vi "Manage Waypoint Shape.vi"(4 "Valid Path?":bool=TRUE, 5 "Draw Arrow":bool, 6 "Coords":cluster{"x":dbl, "y":dbl}, 7 "Drawing Options":T1, 8 "Operation":enum16{"Draw", "Pt Test"}(ring), 9 "new picture in":picture, 10 "Waypoint Position (ft)":cluster{"x":dbl, "y":dbl, "th":dbl}, 11 "Pict Ref":refnum<vi>) -> (0 "Pt Test Results":enum16{"Miss", "Rect Hit", "Arrow Hit"}(ring), 1 "new picture out":picture)   [LabVIEW 2023]
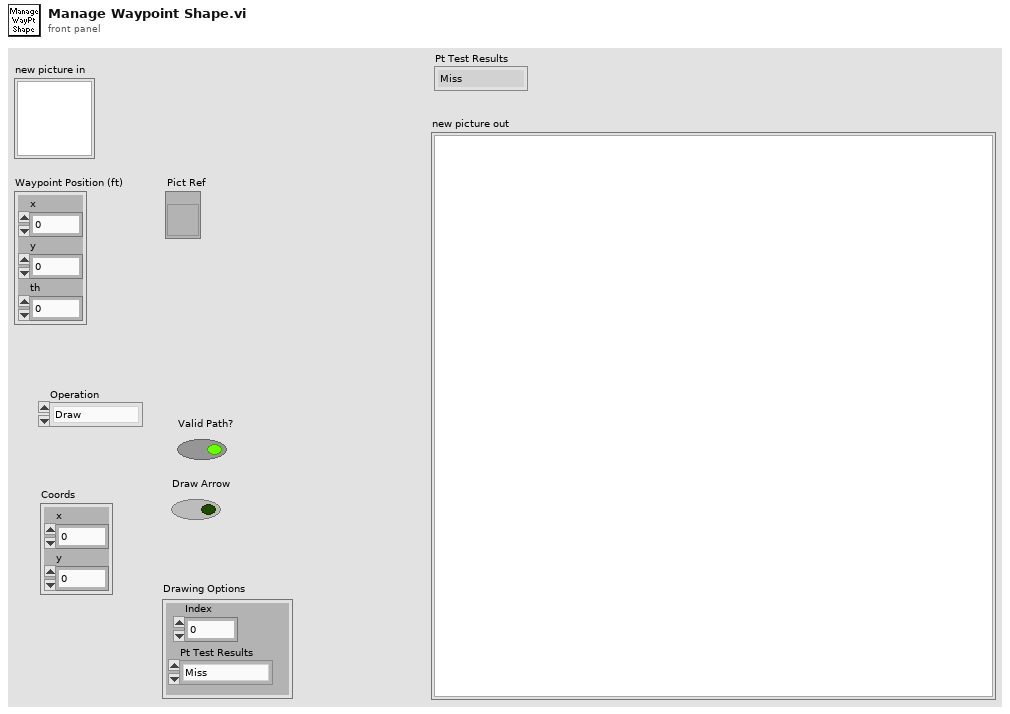
[diagram p1: front panel]
types:
  T1 = cluster{"Index":u32, "Pt Test Results":enum16{"Miss", "Rect Hit", "Arrow Hit"}}
  T2 = typedef "LVPositionTypeDef.ctl" = cluster{"Left":i32, "Top":i32}
  T3 = typedef "LVBoundsTypeDef.ctl" = cluster{"Width":u32, "Height":u32}
  T4 = cluster{"horizontal":enum16{"left", "center", "right"}, "vertical":enum16{"top", "center", "bottom"}}
  T5 = cluster{"Width":u16, "Style":enum32{"Solid", "Dash", "Dot", "DashDot", "DashDotDot"}}
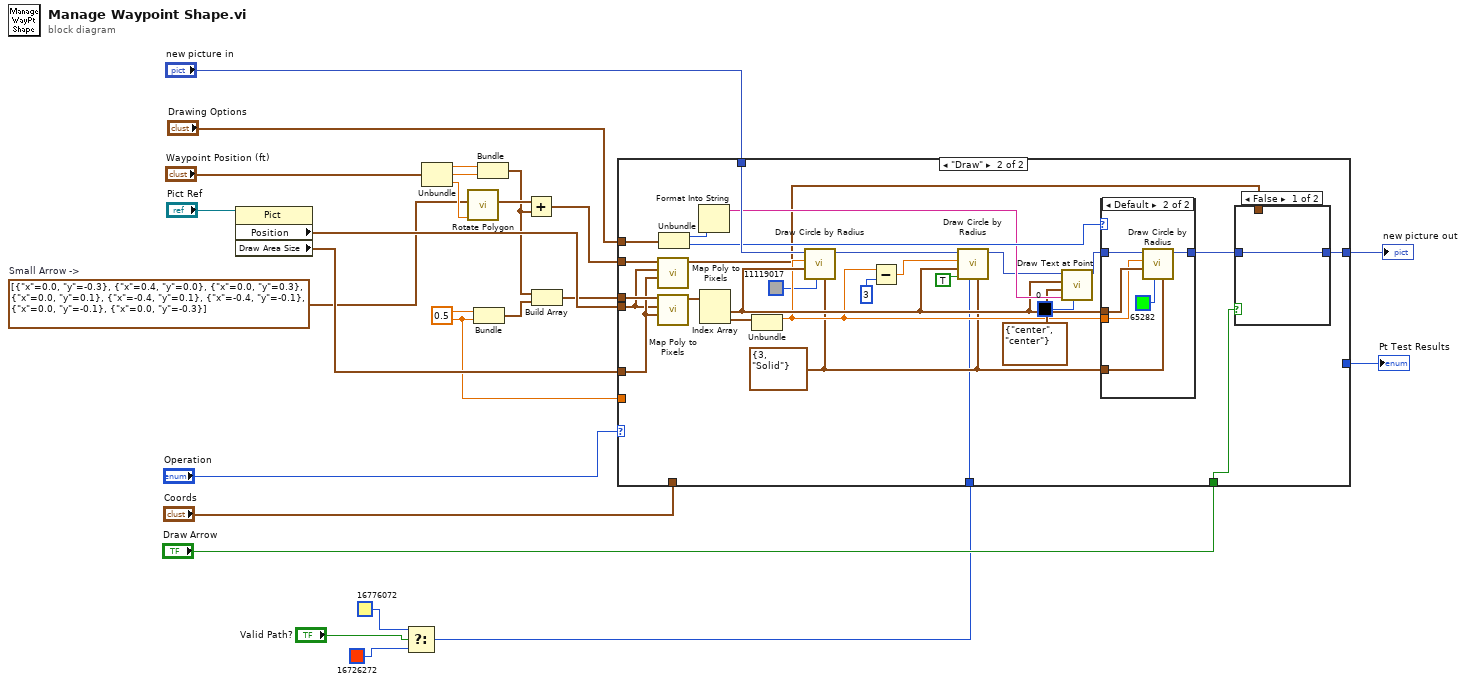
[diagram p0: block diagram]
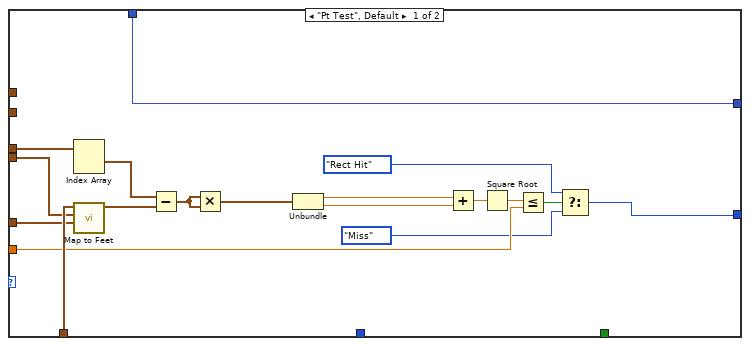
[diagram p2: hidden frame]
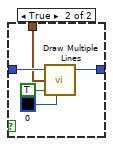
[diagram p3: hidden frame]
diagram:
  w9 = cluster{"x":dbl, "y":dbl}[] [{"x"=0.0, "y"=-0.3}, {"x"=0.4, "y"=0.0}, {"x"=0.0, "y"=0.3}, {"x"=0.0, "y"=0.1}, {"x"=-0.4, "y"=0.1}, {"x"=-0.4, "y"=-0.1}, {"x"=0.0, "y"=-0.1}, {"x"=0.0, "y"=-0.3}]  # Small Arrow ->
  w11 = 0.5 ("y")
  n1 = property on="Property Node" class="Pict"(reference="Pict Ref") -> ("Position"=w20:T2, "Draw Area Size"=w19:T3)  [unwired: 1 in, 2 out]
  n2 = Select(t=u32 16776072 ("color(black)"), s="Valid Path?", f=u32 16726272 ("color(black)")) -> (s? t:f=w1:u32)
  n3 = Unbundle("Waypoint Position (ft)") -> ("x"=w22:dbl, "y"=w23:dbl, "th"=w10:dbl)
  n4 = call "Rotate Polygon.vi"("Angle"=w10, "polygon 2"=w9) -> ("polygon"=w8:cluster{dbl, dbl}[])  [unwired: 9 in]
  n5 = Bundle("y"=w11, "y"=w11) -> (w12:cluster{"y":dbl, "y":dbl})  [unwired: 1 in]
  n6 = Bundle("x"=w22, "y"=w23) -> (w7:cluster{"x":dbl, "y":dbl})  [unwired: 1 in]
  n7 = Add(x=w8, y=w7) -> (x+y=w6:cluster{dbl, dbl}[])
  n8 = Build Array(w7, w12) -> (w13:cluster{"y":dbl, "y":dbl}[])
  n9 = case shown="\"Draw\"" "Operation" {
    tunnel: w13 -> [w38 w69]
    tunnel: [w43 w51] -> w25
    tunnel: "new picture in" -> [w43 w70]
    tunnel: w20 -> [w40 w53]
    tunnel: w19 -> [w41 w54]
    tunnel: "Coords" -> [w42 _]
    tunnel: [w26 _] -> w15
    tunnel: "Drawing Options" -> [_ w71]
    tunnel: w11 -> [w30 _]
    tunnel: w6 -> [_ w55]
    tunnel: "Draw Arrow" -> [_ w45]
    tunnel: w1 -> [_ w46]
    frame "Pt Test", Default {
      n10 = Index Array(array=w38) -> (element #1=w37:cluster{"y":dbl, "y":dbl})  [unwired: 2 in, 1 out]
      n11 = call "Map to Feet.vi"("Draw Area Size"=w41, "Position"=w40, "Coords (px)"=w42) -> ("Point (ft)"=w39:cluster{dbl, dbl})  [unwired: 8 in]
      n12 = Subtract(x=w37, y=w39) -> (x-y=w36:cluster{dbl, dbl})
      n13 = Multiply(x=w36, y=w36) -> (x*y=w35:cluster{dbl, dbl})
      n14 = Unbundle(w35) -> (w34:dbl, w33:dbl)
      n15 = Add(x=w34, y=w33) -> (x+y=w32:dbl)
      n16 = Square Root(x=w32) -> (sqrt(x)=w31:dbl)
      n17 = Less Or Equal?(x=w31, y=w30) -> (x <= y?=w29:bool)
      n18 = Select(t=enum16{"Miss", "Rect Hit", "Arrow Hit"}."Rect Hit" ("Pt Test Results"), s=w29, f=enum16{"Miss", "Rect Hit", "Arrow Hit"}."Miss" ("Pt Test Results")) -> (s? t:f=w26:enum16{"Miss", "Rect Hit", "Arrow Hit"})
    }
    frame "Draw" {
      w49 = T5 {"Width"=3, "Style"=enum."Solid"} ("pen")
      n19 = call "Map Poly to Pixels.vi"("Draw Area Size"=w54, "Position"=w53, "Coords"=w55) -> ("Coords"=w50:cluster{"Horizontal":dbl, "Vertical":dbl}[])  [unwired: 8 in]
      n20 = call "Map Poly to Pixels.vi"("Draw Area Size"=w54, "Position"=w53, "Coords"=w69) -> ("Coords"=w68:cluster{"Horizontal":dbl, "Vertical":dbl}[])  [unwired: 8 in]
      n21 = Unbundle(w71) -> ("Index"=w65:u32, "Pt Test Results"=w66:enum16{"Miss", "Rect Hit", "Arrow Hit"})
      n22 = Format Into String(w65) -> (resulting string=w63:string)  [unwired: 3 in, 1 out]
      n23 = Index Array(array=w68) -> (element #1=w58:cluster{"Horizontal":dbl, "Vertical":dbl}, element #2=w67:cluster{"Horizontal":dbl, "Vertical":dbl})  [unwired: 2 in]
      n24 = Unbundle(w67) -> ("Horizontal"=w57:dbl)  [unwired: 1 out]
      n25 = call <vilib>:"Draw Circle by Radius.vi"("pen"=w49, "color(black)"=u32 11119017, "pixel center"=w58, "radius"=w57, "picture"=w70) -> ("new picture"=w61:picture)  [unwired: 6 in]
      n26 = Subtract(x=w57, y=u16 3 ("Width")) -> (x-y=w44:dbl)
      n27 = call <vilib>:"Draw Circle by Radius.vi"("pen"=w49, "color(black)"=w46, "fill?(F)"=TRUE, "pixel center"=w58, "radius"=w44, "picture"=w61) -> ("new picture"=w60:picture)  [unwired: 5 in]
      n28 = call <vilib>:"Draw Text at Point.vi"("text color(black)"=u32 0, "text"=w63, "alignment(left, top)"=T4 {"horizontal"=enum."center", "vertical"=enum."center"}, "origin"=w58, "picture"=w60) -> ("new picture"=w64:picture)  [unwired: 5 in, 1 out]
      n29 = case shown="Default" w66 {
        tunnel: w64 -> [w78 w84]
        tunnel: [w78 w83] -> w52
        tunnel: w58 -> [_ w82]
        tunnel: w57 -> [_ w81]
        tunnel: w49 -> [_ w79]
        frame "Miss" {
        }
        frame Default {
          n30 = call <vilib>:"Draw Circle by Radius.vi"("pen"=w79, "color(black)"=u32 65282, "pixel center"=w82, "radius"=w81, "picture"=w84) -> ("new picture"=w83:picture)  [unwired: 6 in]
        }
      }
      n31 = case shown="False" w45 {
        tunnel: w52 -> [w72 w77]
        tunnel: [w72 w76] -> w51
        tunnel: w50 -> [_ w75]
        frame False {
        }
        frame True {
          n32 = call <vilib>:"Draw Multiple Lines.vi"("picture"=w77, "line endpoints"=w75, "fill?(F)"=TRUE, "color(black)"=u32 0) -> ("new picture"=w76:picture)  [unwired: 5 in]
        }
      }
    }
  }
  "new picture out" <- w25
  "Pt Test Results" <- w15
